vi "Proxy - Dist Set LLB Caching.vi"(8 "error in (no error)":errorcluster, 11 "enable?":bool) -> (0 "error out":errorcluster)   [LabVIEW 2009]
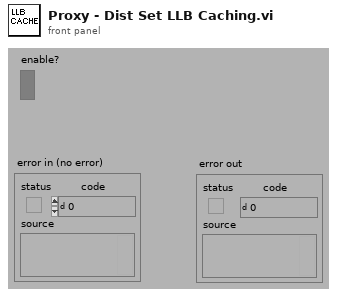
[diagram p1: front panel]
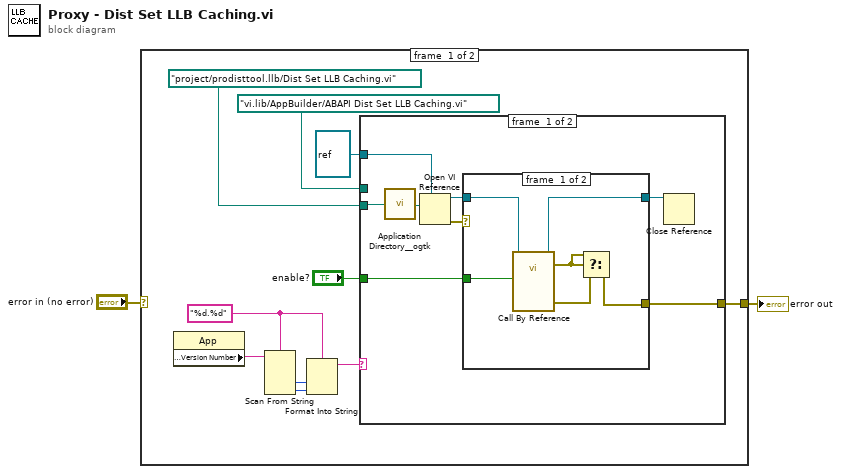
[diagram p0: block diagram]
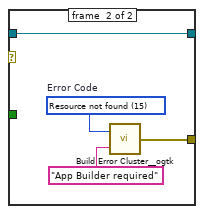
[diagram p2: hidden frame]
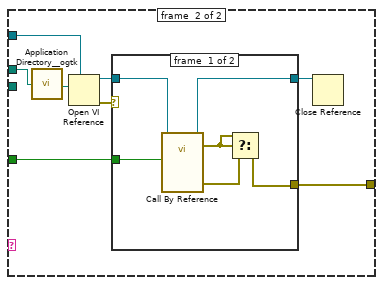
[diagram p3: hidden frame]
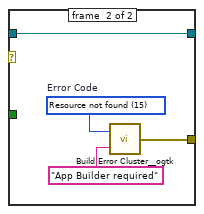
[diagram p4: hidden frame]
diagram:
  n1 = case shown="No Error" "error in (no error)" {
    selector: "error in (no error)" -> [_ w49]
    tunnel: [w4 w49] -> w1
    frame #0 {
      w11 = "%d.%d" ("format string")
      n2 = property class="App"() -> ("Application:Version Number"=w12:string)  [unwired: 2 in, 2 out]
      n3 = Scan From String(format string=w11, input string=w12) -> (output 1=w10:i32, output 2=w9:i32)  [unwired: 4 in, 3 out]
      n4 = Format Into String(format string=w11, w10, w9) -> (resulting string=w8:string)  [unwired: 2 in, 1 out]
      n5 = case shown="\"8.0\", Default" w8 {
        tunnel: path "project/prodisttool.llb/Dist Set LLB Caching.vi" ("Relative path (.)") -> [w16 _]
        tunnel: [w19 w37] -> w4
        tunnel: path "vi.lib/AppBuilder/ABAPI Dist Set LLB Caching.vi" ("Relative path (.)") -> [_ w32]
        tunnel: "enable?" -> [w14 w33]
        tunnel: refnum<vi> refnum ("LV 6.1/7.0/7.1/8.0 VI Refnum (for type)") -> [w13 w31]
        frame #0 {
          n6 = call <userlib>:"Application Directory__ogtk.vi"("Relative path (.)"=w16) -> ("Application Directory (+ Relative)"=w15:path)
          n7 = Open VI Reference(type specifier VI Refnum (for type only)=w13, vi path=w15) -> (vi reference=w18:refnum<vi>, error out=w20:errorcluster)  [unwired: 4 in]
          n8 = case shown="No Error" w20 {
            tunnel: [w25 w29] -> w19
            tunnel: w18 -> [w24 w28]
            tunnel: [w22 w28] -> w17
            tunnel: w14 -> [w21 _]
            frame #0 {
              n9 = call-by-ref "?"(reference=w24, "enable?"=w21) -> (reference out=w22:refnum<vi>, error out=w26:errorcluster, "error out"=w23:errorcluster)  [unwired: 11 in]
              n10 = Select(t=w26, s=w26, f=w23) -> (s? t:f=w25:errorcluster)
            }
            frame #1 {
              w27 = u16 15 items=["No error", "Argument error", "Memory is full", "Out of zone", "End of file", "File already open", "Generic file I/O error", "File not found", "File permission error", "Disk is full", "Duplicate path", "Too many files open", "System feature not enabled", "Resource file not found", "Cannot add resource", "Resource not found", "Image not found", "Image memory error", "Pen does not exist", "Config type invalid", "Config token not found", "Config parse error", "Config memory error", "Bad external code format", "Bad external code offset", "External code not present", "Null window", "Destroy window error", "Null menu", "Print aborted", "Bad print record", "Print driver error", "Windows error during printing", "Memory error during printing", "Print dialog error", "Generic print error", "Invalid device refnum", "Device not found", "Device parameter error", "Device unit error", "Cannot open device", "Device call aborted", "Generic error", "Cancelled by user", "Object ID too low", "Object ID too high", "Object not in heap", "Unknown heap", "Unknown object (invalid DefProc)", "Unknown object (DefProc not in table)", "Message out of range", "Invalid (null) method", "Unknown message", "Manager call not supported", "Bad address", "Network operation in progress", "Network operation timed out", "Connection is busy", "Network attribute not supported", "Network error", "Address in use", "System out of memory", "Connection aborted", "Connection refused", "Not connected", "Already connected", "Connection closed", "Initialization error (interapplication manager)", "Bad occurrence", "Wait on unbound occurrence handler", "Occurrence queue overflow", "Datalog type conflict", "Unused", "Unrecognized type (interapplication manager)", "Memory corrupt", "Failed to make temporary DLL", "Old CIN version", "Drag socket not found", "Failed to load drop-object", "Failed to register OLE object", "Failed to release OLE object", "Format specifier type mismatch", "Unknown format specifier", "Too few format specifiers", "Too many format specifiers", "Scan failed", "Newer CIN version", "OLE Convert", "Runtime menu error", "Password tampered", "Unknown error code"]  # Error Code
              n11 = call <userlib>:"Build Error Cluster__ogtk.vi"("String to Prepend to source (\"\")"="App Builder required" ("String to Prepend to source (\"\")"), "code"=w27) -> ("error out"=w29:errorcluster)
            }
          }
          n12 = Close Reference(reference=w17) -> ()  [unwired: 1 in, 1 out]
        }
        frame #1 {
          n13 = call <userlib>:"Application Directory__ogtk.vi"("Relative path (.)"=w32) -> ("Application Directory (+ Relative)"=w34:path)
          n14 = Open VI Reference(type specifier VI Refnum (for type only)=w31, vi path=w34) -> (vi reference=w36:refnum<vi>, error out=w38:errorcluster)  [unwired: 4 in]
          n15 = case shown="No Error" w38 {
            tunnel: [w43 w47] -> w37
            tunnel: w36 -> [w42 w46]
            tunnel: [w40 w46] -> w35
            tunnel: w33 -> [w39 _]
            frame #0 {
              n16 = call-by-ref "?"(reference=w42, "enable?"=w39) -> (reference out=w40:refnum<vi>, error out=w44:errorcluster, "error out"=w41:errorcluster)  [unwired: 11 in]
              n17 = Select(t=w44, s=w44, f=w41) -> (s? t:f=w43:errorcluster)
            }
            frame #1 {
              w45 = u16 15 items=["No error", "Argument error", "Memory is full", "Out of zone", "End of file", "File already open", "Generic file I/O error", "File not found", "File permission error", "Disk is full", "Duplicate path", "Too many files open", "System feature not enabled", "Resource file not found", "Cannot add resource", "Resource not found", "Image not found", "Image memory error", "Pen does not exist", "Config type invalid", "Config token not found", "Config parse error", "Config memory error", "Bad external code format", "Bad external code offset", "External code not present", "Null window", "Destroy window error", "Null menu", "Print aborted", "Bad print record", "Print driver error", "Windows error during printing", "Memory error during printing", "Print dialog error", "Generic print error", "Invalid device refnum", "Device not found", "Device parameter error", "Device unit error", "Cannot open device", "Device call aborted", "Generic error", "Cancelled by user", "Object ID too low", "Object ID too high", "Object not in heap", "Unknown heap", "Unknown object (invalid DefProc)", "Unknown object (DefProc not in table)", "Message out of range", "Invalid (null) method", "Unknown message", "Manager call not supported", "Bad address", "Network operation in progress", "Network operation timed out", "Connection is busy", "Network attribute not supported", "Network error", "Address in use", "System out of memory", "Connection aborted", "Connection refused", "Not connected", "Already connected", "Connection closed", "Initialization error (interapplication manager)", "Bad occurrence", "Wait on unbound occurrence handler", "Occurrence queue overflow", "Datalog type conflict", "Unused", "Unrecognized type (interapplication manager)", "Memory corrupt", "Failed to make temporary DLL", "Old CIN version", "Drag socket not found", "Failed to load drop-object", "Failed to register OLE object", "Failed to release OLE object", "Format specifier type mismatch", "Unknown format specifier", "Too few format specifiers", "Too many format specifiers", "Scan failed", "Newer CIN version", "OLE Convert", "Runtime menu error", "Password tampered", "Unknown error code"]  # Error Code
              n18 = call <userlib>:"Build Error Cluster__ogtk.vi"("String to Prepend to source (\"\")"="App Builder required" ("String to Prepend to source (\"\")"), "code"=w45) -> ("error out"=w47:errorcluster)
            }
          }
          n19 = Close Reference(reference=w35) -> ()  [unwired: 1 in, 1 out]
        }
      }
    }
    frame #1 {
    }
  }
  "error out" <- w1
